vi "Upload_To_ADAM_Server.vi"(0 "Channel Names":string[](array[string]), 1 "Averaging Period (s)":dbl=1.0, 2 "Channel Values":dbl[](array[numeric]), 3 "Shift In":dbl[](array[numeric]), 4 "First Loop":bool) -> (5 "Shift Out":dbl[](array[numeric]))   [LabVIEW 2010]
uses:
  ADAM Controls/Update_scan_value.ctl
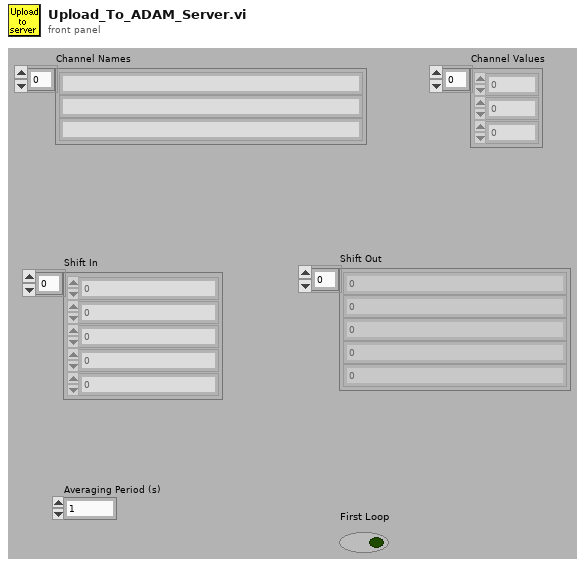
[diagram p1: front panel]
types:
  T1 = typedef "Update_scan_value.ctl" = cluster{"Channel Name":string, "New Value":dbl}
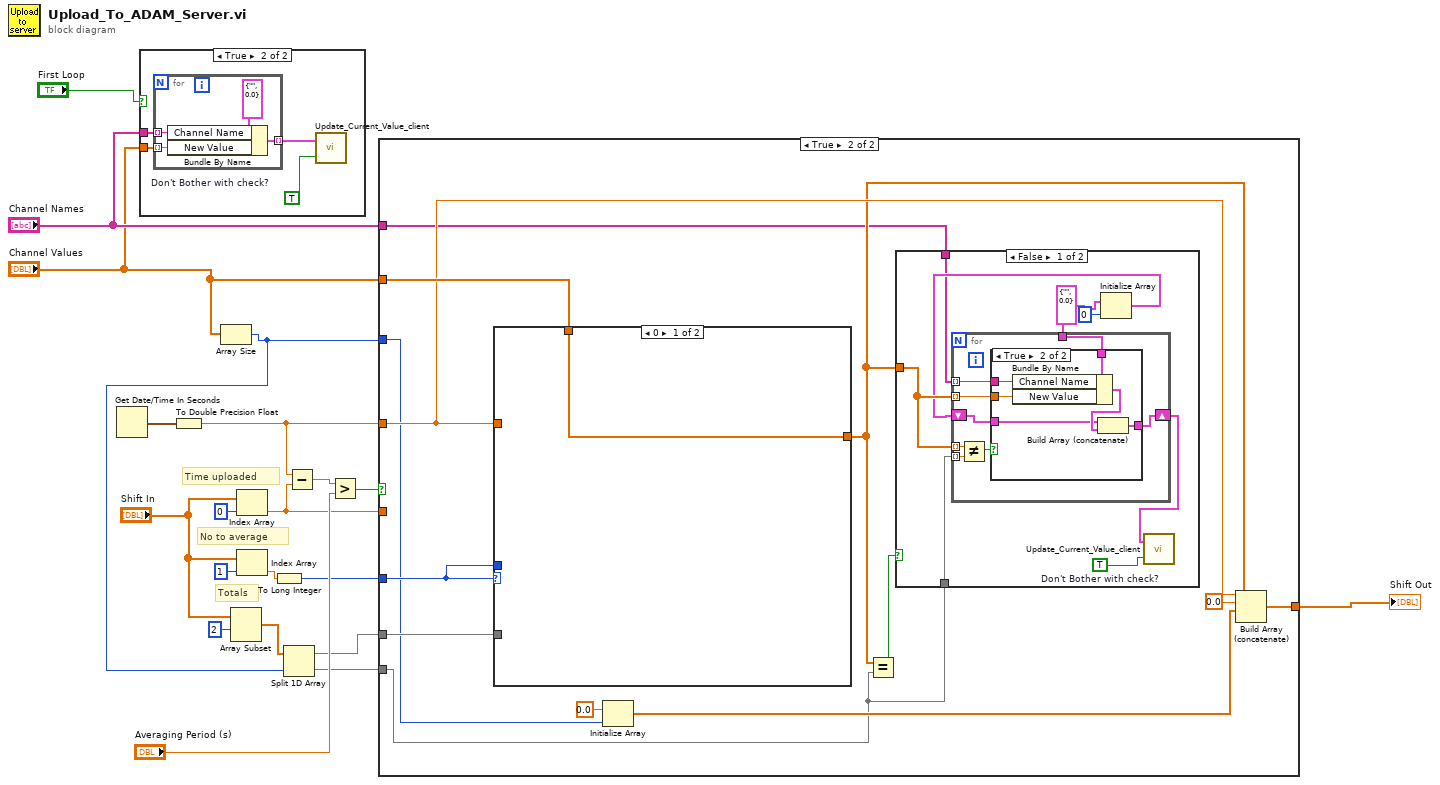
[diagram p0: block diagram]
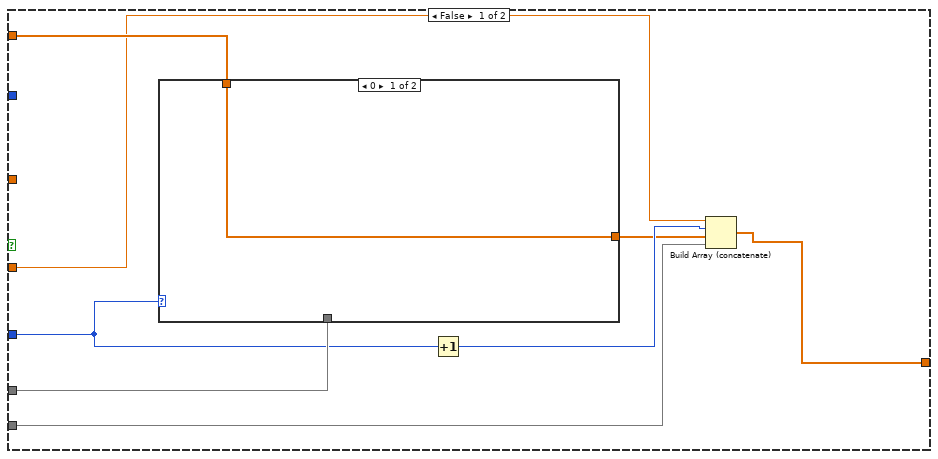
[diagram p3: hidden frame]
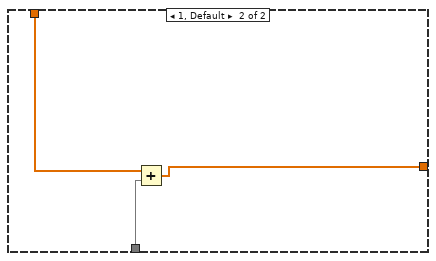
[diagram p4: hidden frame]
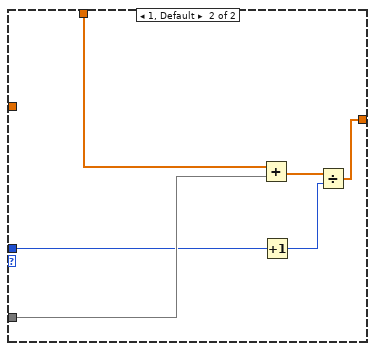
[diagram p7: hidden frame]
diagram:
  # "Totals"
  # "No to average"
  # "Time uploaded"
  n1 = Get Date/Time In Seconds() -> (seconds since 1Jan1904=w19:timestamp)
  n2 = case shown="True" "First Loop" {
    tunnel: "Channel Names" -> [_ w22]
    tunnel: "Channel Values" -> [_ w21]
    frame False {
    }
    frame True {
      w24 = TRUE  # Don't Bother with check?
      n3 = for {
        tunnel: [w27] -> w23 mode=indexing
        tunnel: w22 -> [w26] mode=indexing
        tunnel: w21 -> [w25] mode=indexing
        n4 = Bundle By Name(cluster=T1 {"Channel Name"="", "New Value"=0.0} ("Update Scan Value Cluster"), "Channel Name"=w26, "New Value"=w25) -> (w27:T1)
      }
      n5 = call "Update_Current_Value_client.vi"("Don't Bother with check?"=w24, "Update array in"=w23) -> ()
    }
  }
  n6 = To Double Precision Float(number=w19) -> (double precision float=w10:dbl)
  n7 = Array Size(array="Channel Values") -> (size(s)=w6:i32)
  n8 = Array Subset(array="Shift In", index=2) -> (w7:dbl[])  [unwired: 1 in]
  n9 = Index Array(array="Shift In", index=0) -> (element=w8:dbl)
  n10 = Index Array(array="Shift In", index=1) -> (element=w12:dbl)
  n11 = To Long Integer(number=w12) -> (32bit integer=w11:i32)
  n12 = Split 1D Array(array=w7, index=w6) -> (first subarray=w5:dbl[], second subarray=w4:dbl[])
  n13 = Subtract(x=w10, y=w8) -> (x-y=w18:dbl)
  n14 = Greater?(x=w18, y="Averaging Period (s)") -> (0:w16:bool)
  n15 = case shown="True" w16 {
    tunnel: "Channel Values" -> [w36 w53]
    tunnel: w5 -> [w35 w48]
    tunnel: w11 -> [w33 w52]
    tunnel: w10 -> [_ w51]
    tunnel: [w30 w49] -> w9
    tunnel: w8 -> [w34 _]
    tunnel: w6 -> [_ w45]
    tunnel: w4 -> [w29 w42]
    tunnel: "Channel Names" -> [_ w41]
    frame False {
      n16 = case shown="0" w33 {
        tunnel: w36 -> [w37 w40]
        tunnel: w35 -> [_ w39]
        tunnel: [w37 w38] -> w31
        frame 0 {
        }
        frame 1, Default {
          n17 = Add(x=w40, y=w39) -> (x+y=w38:dbl[])
        }
      }
      n18 = Increment(x=w33) -> (x+1=w32:i32)
      n19 = Build Array (concatenate)(w34, w32, w31, w29) -> (w30:dbl[])
    }
    frame True {
      n20 = case shown="0" w52 {
        tunnel: w51 -> [_ _]
        tunnel: w48 -> [_ w82]
        tunnel: w53 -> [w77 w83]
        tunnel: w52 -> [_ w81]
        tunnel: [w77 w78] -> w44
        frame 0 {
        }
        frame 1, Default {
          n21 = Add(x=w83, y=w82) -> (x+y=w80:dbl[])
          n22 = Increment(x=w81) -> (x+1=w79:i32)
          n23 = Divide(x=w80, y=w79) -> (x/y=w78:dbl[])
        }
      }
      n24 = Initialize Array(0.0 ("element"), w45) -> (w46:dbl[])
      n25 = Equal?(x=w44, y=w42) -> (x = y?=w43:bool)
      n26 = case shown="False" w43 {
        tunnel: w44 -> [w60 _]
        tunnel: w42 -> [w59 _]
        tunnel: w41 -> [w54 _]
        frame False {
          w61 = TRUE  # Don't Bother with check?
          w58 = T1 {"Channel Name"="", "New Value"=0.0} ("Update Scan Value Cluster")
          n27 = Initialize Array(w58, 0 ("dimension size")) -> (w56:T1[])
          n28 = for {
            tunnel: w58 -> [w69]
            tunnel: w54 -> [w68] mode=indexing
            tunnel: w60 -> [w67] mode=indexing
            shift-right: [w63] -> w55
            shift-left: w56 -> [w64]
            tunnel: w60 -> [w66] mode=indexing
            tunnel: w59 -> [w65] mode=indexing
            n29 = Not Equal?(x=w66, y=w65) -> (x != y?=w62:bool)
            n30 = case shown="True" w62 {
              tunnel: w69 -> [_ w76]
              tunnel: w68 -> [_ w75]
              tunnel: w67 -> [_ w74]
              tunnel: w64 -> [w70 w72]
              tunnel: [w70 w71] -> w63
              frame False {
              }
              frame True {
                n31 = Bundle By Name(cluster=w76, "Channel Name"=w75, "New Value"=w74) -> (w73:T1)
                n32 = Build Array (concatenate)(w72, w73) -> (w71:T1[])
              }
            }
          }
          n33 = call "Update_Current_Value_client.vi"("Don't Bother with check?"=w61, "Update array in"=w55) -> ()
        }
        frame True {
        }
      }
      n34 = Build Array (concatenate)(w51, 0.0 ("element"), w46, w44) -> (w49:dbl[])
    }
  }
  "Shift Out" <- w9
